vi "Get Controller Card Model.vi"(11 "controllerCardModel":string) -> (2 "function return":u32, 3 "controllerCardModel out":string)   [LabVIEW 2018, in "Copy of Andor SDK.lvlib"]
doc: "EXPNETTYPE unsigned int WINAPI GetControllerCardModel(char * controllerCardModel);"
uses:
  Copy of Andor SDK.lvlib
  <userlib>/Andor SDK/ATMCD32D.dll
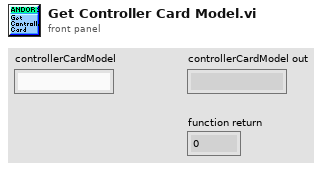
[diagram p1: front panel]
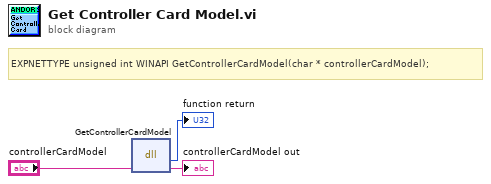
[diagram p0: block diagram]
diagram:
  # "EXPNETTYPE unsigned int WINAPI GetControllerCardModel(char * controllerCardModel);"
  n1 = dll-call lib="C:/Program Files (x86)/National Instruments/LabVIEW 2018/user.lib/Andor SDK/ATMCD32D.*" fn="GetControllerCardModel"("controllerCardModel"="controllerCardModel") -> (→"function return":u32, "controllerCardModel"=→"controllerCardModel out":string)  [unwired: 3 in, 2 out]
